vi "IMU Get Yaw Landscapevi.vi"(8 "error in (no error)":errorcluster) -> (0 "error out":errorcluster, 2 "timestamp out":i64, 3 "yaw":dbl(graph))   [LabVIEW 2026, in "MrcLib.lvlib"]
doc: "Return the computed Yaw of the built-in sensor assuming it is mounted vertically with long edge parallel to the ground (somewhat common)."
uses:
  MrcLib.lvlib
  <vilib>/MRC/MrcLib/VIs/IMU/MRC IMU Get Yaw Landscape.vi
panel:
  out "yaw out":dbl
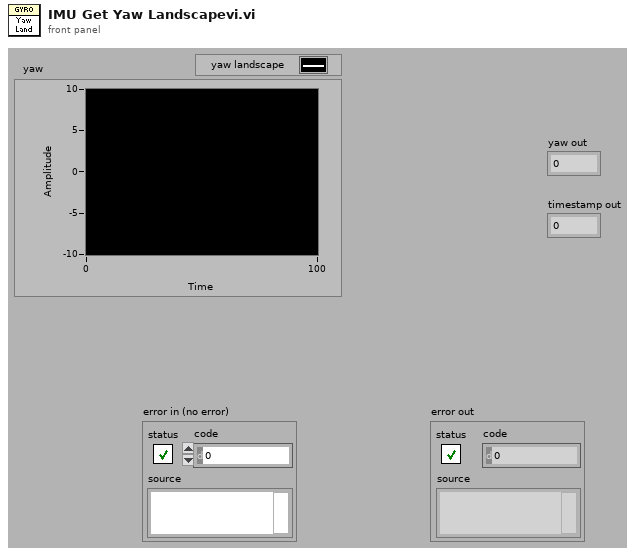
[diagram p1: front panel]
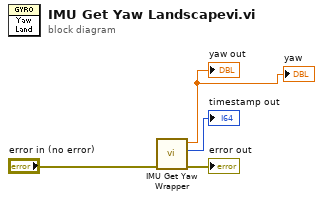
[diagram p0: block diagram]
diagram:
  n1 = call-poly "IMU Get Yaw Wrapper.vi"("error in (no error)"="error in (no error)") -> ("error out"=→"error out":errorcluster, "timestamp out"=→"timestamp out":i64, "yaw out"=→"yaw out" →"yaw":dbl)  [unwired: 7 in, 1 out]
